vi "10-tap-lp.vi"(10 "Input":dbl[](array[numeric])) -> (2 "Output Array":dbl[](array[numeric]))   [LabVIEW 2015]
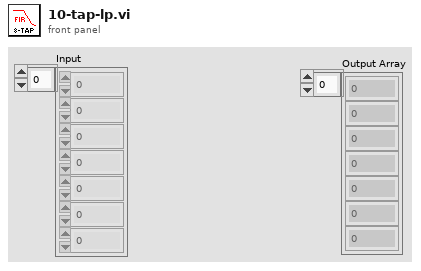
[diagram p1: front panel]
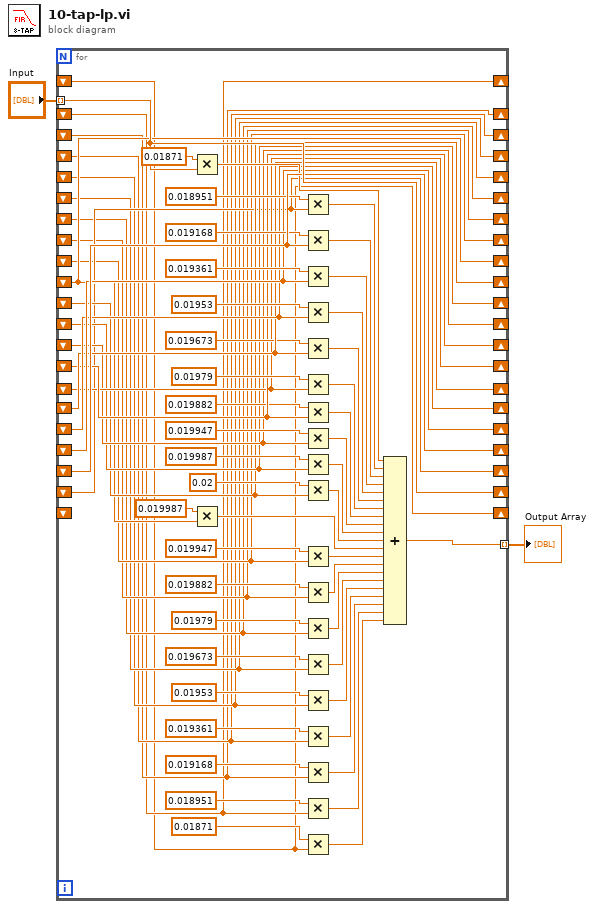
[diagram p0: block diagram]
diagram:
  n1 = for {
    tunnel: "Input" -> [w66] mode=indexing
    shift-right: [w66] -> _
    shift-left: _ -> [w29]
    shift-right: [w29] -> _
    shift-left: _ -> [w65]
    shift-right: [w65] -> _
    shift-left: _ -> [w56]
    tunnel: [w28] -> w1 mode=indexing
    shift-right: [w56] -> _
    shift-left: _ -> [w53]
    shift-right: [w53] -> _
    shift-left: _ -> [w52]
    shift-right: [w52] -> _
    shift-left: _ -> [w44]
    shift-right: [w44] -> _
    shift-left: _ -> [w47]
    shift-right: [w47] -> _
    shift-left: _ -> [w41]
    shift-right: [w41] -> _
    shift-left: _ -> [w39]
    shift-right: [w39] -> _
    shift-left: _ -> [w37]
    shift-right: [w37] -> _
    shift-left: _ -> [w32]
    shift-right: [w32] -> _
    shift-left: _ -> [w27]
    shift-right: [w27] -> _
    shift-left: _ -> [w24]
    shift-right: [w24] -> _
    shift-left: _ -> [w21]
    shift-right: [w21] -> _
    shift-left: _ -> [w19]
    shift-right: [w19] -> _
    shift-left: _ -> [w11]
    shift-right: [w11] -> _
    shift-left: _ -> [w10]
    shift-right: [w10] -> _
    shift-left: _ -> [w9]
    shift-right: [w9] -> _
    shift-left: _ -> [w8]
    shift-right: [w8] -> _
    shift-left: _ -> [w7]
    shift-right: [w7] -> _
    shift-left: _ -> [_]
    n2 = Multiply(x=0.01871, y=w66) -> (x*y=w64:dbl)
    n3 = Multiply(x=0.019987, y=w32) -> (x*y=w33:dbl)
    n4 = Multiply(x=0.018951, y=w29) -> (x*y=w63:dbl)
    n5 = Multiply(x=0.019168, y=w65) -> (x*y=w62:dbl)
    n6 = Multiply(x=0.019361, y=w56) -> (x*y=w61:dbl)
    n7 = Multiply(x=0.01953, y=w53) -> (x*y=w54:dbl)
    n8 = Multiply(x=0.019673, y=w52) -> (x*y=w49:dbl)
    n9 = Multiply(x=0.01979, y=w44) -> (x*y=w48:dbl)
    n10 = Multiply(x=0.019882, y=w47) -> (x*y=w43:dbl)
    n11 = Multiply(x=0.019947, y=w41) -> (x*y=w42:dbl)
    n12 = Multiply(x=0.019987, y=w39) -> (x*y=w35:dbl)
    n13 = Multiply(x=0.02, y=w37) -> (x*y=w34:dbl)
    n14 = Multiply(x=0.019947, y=w27) -> (x*y=w30:dbl)
    n15 = Multiply(x=0.019882, y=w24) -> (x*y=w25:dbl)
    n16 = Multiply(x=0.01979, y=w21) -> (x*y=w22:dbl)
    n17 = Multiply(x=0.019673, y=w19) -> (x*y=w18:dbl)
    n18 = Multiply(x=0.01953, y=w11) -> (x*y=w16:dbl)
    n19 = Multiply(x=0.019361, y=w10) -> (x*y=w6:dbl)
    n20 = Multiply(x=0.019168, y=w9) -> (x*y=w5:dbl)
    n21 = Multiply(x=0.018951, y=w8) -> (x*y=w4:dbl)
    n22 = Multiply(x=0.01871, y=w7) -> (x*y=w3:dbl)
    n23 = Compound Arithmetic op=ADD(w64, w63, w62, w61, w54, w49, w48, w43, w42, w35, w34, w33, w30, w25, w22, w18, w16, w6, w5, w4, w3) -> (w28:dbl)
  }
  "Output Array" <- w1
